vi "Read Monitor Channel.vi"(8 "error in":errorcluster, 10 "channel number in":u8, 11 "board handle in":u8) -> (0 "error out":errorcluster, 1 "monitor data out":T1[](array[typedef]), 2 "channel number out":u8, 3 "board handle out":u8)   [LabVIEW 2020, in "AIM ARINC 429 Hardware API.lvlib"]
uses:
  AIM ARINC 429 Hardware API.lvlib
  <instrlib>/AIM GmbH/_ARINC-429/AIM429LV.lvlib
  Monitor Data.ctl
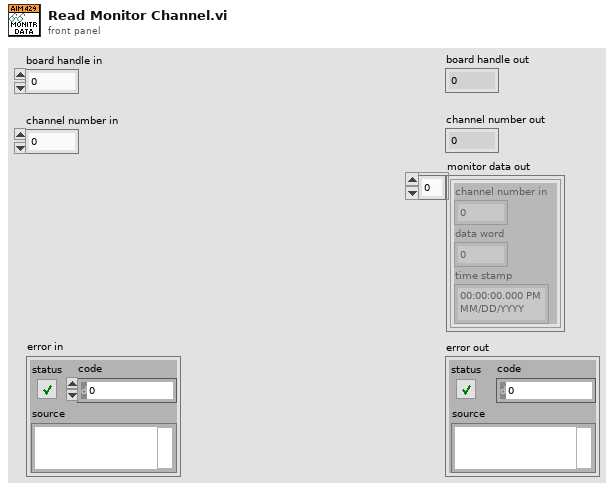
[diagram p1: front panel]
types:
  T1 = typedef "AIM ARINC 429 Hardware API.lvlib/Monitor Data.ctl" = cluster{"channel number in":u8, "data word":u32, "time stamp":timestamp}
  T2 = typedef "AIM429LV.lvlib/rx_stack_entry.ctl" = cluster{"label data":u32, "time tag":u32, "buffer report word":u32, "day of year":u32}
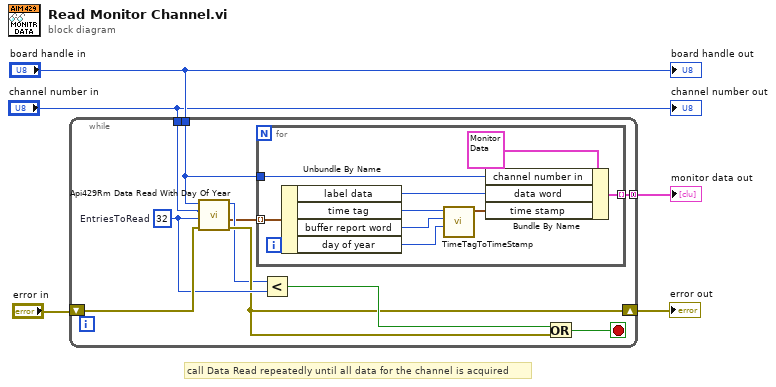
[diagram p0: block diagram]
diagram:
  # "call Data Read repeatedly until all data for the channel is acquired"
  n1 = while {
    tunnel: "board handle in" -> [w7]
    tunnel: "channel number in" -> [w13]
    shift-right: [w10] -> w2
    shift-left: "error in" -> [w12]
    tunnel: [w6] -> w1 mode=concatenating
    stop <- w14 stop-if-true
    w11 = u16 32  # EntriesToRead
    n2 = call <instrlib>:"Api429Rm Data Read With Day Of Year.vi"("error in"=w12, "uw_EntriesToRead"=w11, "b_Chn"=w13, "board_handle"=w7) -> ("error out"=w10:errorcluster, "px_SData"=w8:T2[], "puw_Count"=w9:u16)  [unwired: 5 in]
    n3 = for {
      tunnel: w8 -> [w24] mode=indexing
      tunnel: w7 -> [w19]
      tunnel: [w16] -> w6 mode=indexing
      n4 = Unbundle By Name(w24) -> ("label data"=w17:u32, "time tag"=w23:u32, "buffer report word"=w22:u32, "day of year"=w21:u32)
      n5 = call <instrlib>:"TimeTagToTimeStamp.vi"("day of year"=w21, "buffer report word"=w22, "time tag"=w23) -> ("time stamp"=w18:timestamp)  [unwired: 7 in, 1 out]
      n6 = Bundle By Name(cluster=T1 {"channel number in"=0, "data word"=0, "time stamp"=timestamp(0 s since 1904-01-01)} ("Word"), "channel number in"=w19, "data word"=w17, "time stamp"=w18) -> (w16:T1)
    }
    n7 = Less?(x=w9, y=w11) -> (x < y?=w15:bool)
    n8 = Or(x=w15, y=w10) -> (x .or. y?=w14:bool)
  }
  "error out" <- w2
  "monitor data out" <- w1
  "board handle out" <- "board handle in"
  "channel number out" <- "channel number in"
